vi "readFromXML.vi"(8 "error in (no error)":errorcluster, 10 "XML in":string, 11 "AzCurrentWrap in":refnum<class "AzCurrentWrap.lvclass">) -> (0 "error out":errorcluster, 3 "AzCurrentWrap out":refnum<class "AzCurrentWrap.lvclass">)   [LabVIEW 2022 SP3, in "TCSDataDefinitions.lvlib" / "TCSCommand.lvlib" / "CableWrapCommands.lvlib" / "AzCurrentWrap.lvclass"]
uses:
  AzCurrentWrap.lvclass
  CableWrapCommands/CableWrapCommands.lvclass
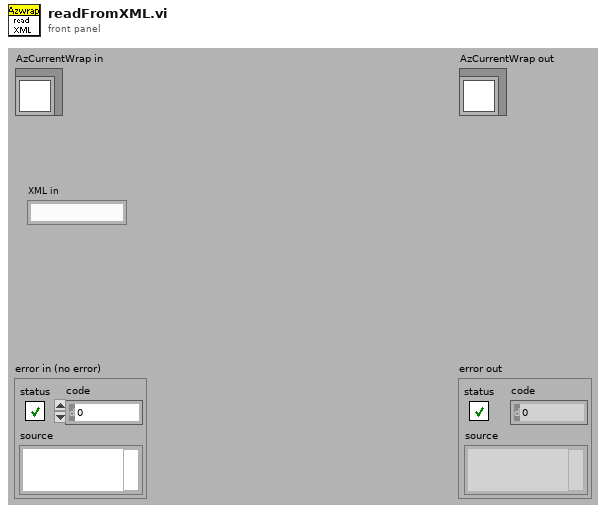
[diagram p1: front panel]
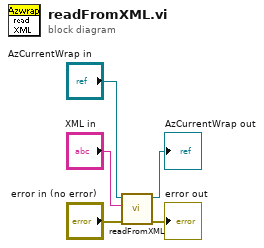
[diagram p0: block diagram]
diagram:
  n1 = call-parent "readFromXML.vi"("error in (no error)"="error in (no error)", "XML in"="XML in", "CableWrapCommands in"="AzCurrentWrap in") -> ("error out"=→"error out":errorcluster, "CableWrapCommands out"=→"AzCurrentWrap out":refnum<class "AzCurrentWrap.lvclass">)  [unwired: 7 out]
